vi "P2_Contador99.vi"() -> ()   [LabVIEW 2020]
panel:
  out "a 2":bool
  out "f":bool
  out "e":bool
  out "b":bool
  out "a":bool
  out "b 2":bool
  out "c 2":bool
  out "d 2":bool
  out "g 2":bool
  out "f 2":bool
  out "e 2":bool
  out "c":bool
  out "d":bool
  out "g":bool
  in  "?":bool
  in  "?":bool
  # "Ascendente"
  # "Descendente"
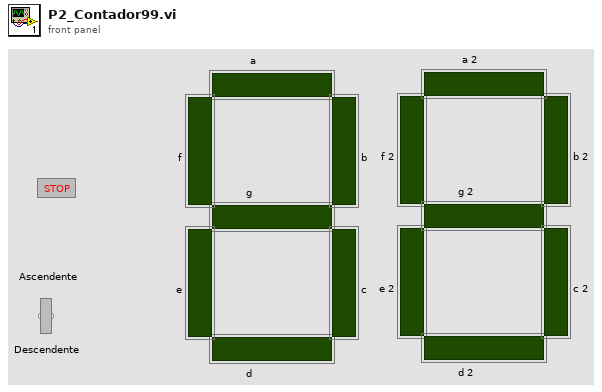
[diagram p1: front panel]
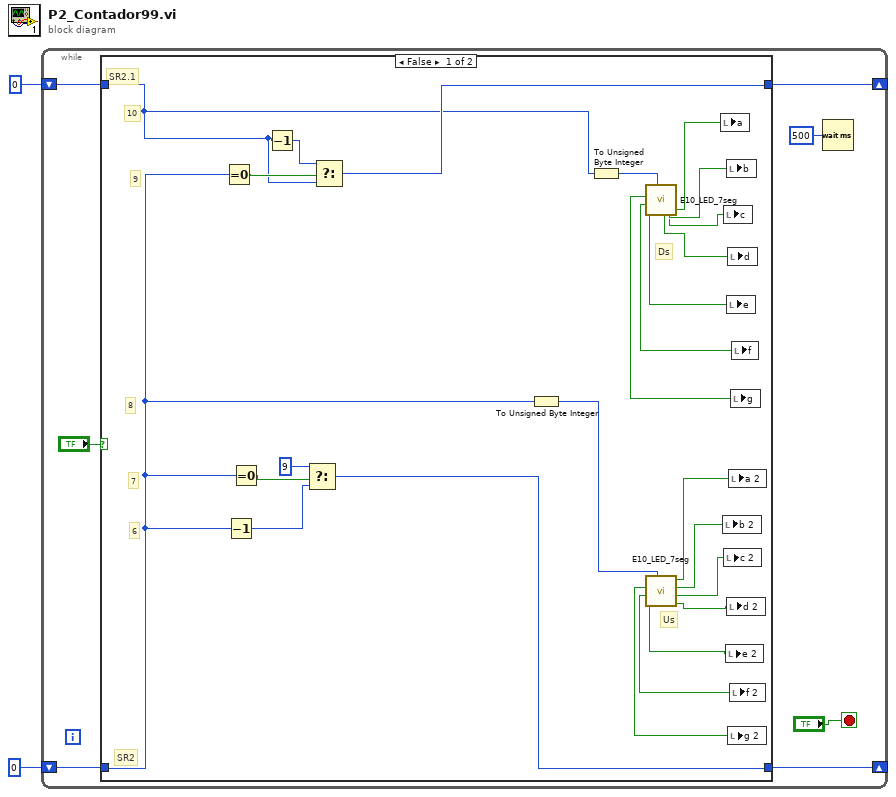
[diagram p0: block diagram]
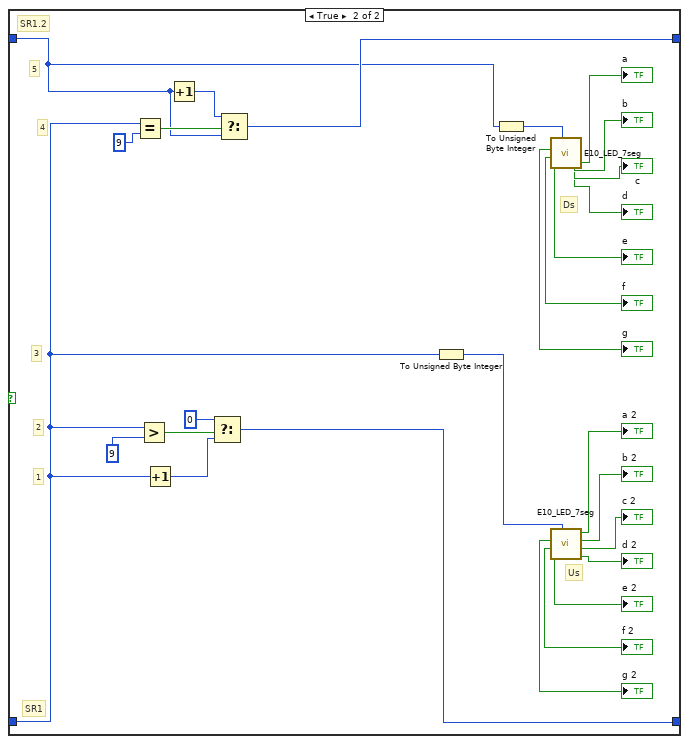
[diagram p2: hidden frame]
diagram:
  n1 = while {
    shift-right: [w8] -> _
    shift-left: 0 -> [w7]
    shift-right: [w5] -> _
    shift-left: 0 -> [w6]
    stop <- "?" stop-if-true
    n2 = case shown="False" "?" {
      tunnel: [w31 w44] -> w8
      tunnel: w7 -> [w11 w37]
      tunnel: w6 -> [w10 w35]
      tunnel: [w13 w36] -> w5
      frame False {
        # "SR2.1"
        # "SR2"
        # "10"
        # "9"
        # "8"
        # "7"
        # "6"
        # "Ds"
        # "Us"
        n3 = Equal To 0?(x=w11) -> (x = 0?=w29:bool)
        n4 = Decrement(x=w11) -> (x-1=w28:i32)
        n5 = Equal To 0?(x=w11) -> (x = 0?=w30:bool)
        n6 = Decrement(x=w10) -> (x-1=w12:i32)
        n7 = Select(t=9, s=w30, f=w28) -> (s? t:f=w31:i32)
        n8 = Select(t=w12, s=w29, f=w10) -> (s? t:f=w13:i32)
        n9 = To Unsigned Byte Integer(number=w11) -> (unsigned 8bit integer=w33:u8)
        n10 = To Unsigned Byte Integer(number=w10) -> (unsigned 8bit integer=w34:u8)
        n11 = call "E10_LED_7seg.vi"("Numeric"=w34) -> ("d"=w24:bool, "c"=w25:bool, "b"=w26:bool, "a"=w27:bool, "e"=w23:bool, "f"=w22:bool, "g"=w21:bool)  [unwired: 1 in]
        n12 = call "E10_LED_7seg.vi"("Numeric"=w33) -> ("d"=w17:bool, "c"=w18:bool, "b"=w19:bool, "a"=w20:bool, "e"=w16:bool, "f"=w15:bool, "g"=w14:bool)  [unwired: 1 in]
        n13 = local write "a"(w27) -> ()
        n14 = local write "b 2"(w19) -> ()
        n15 = local write "c"(w25) -> ()
        n16 = local write "c 2"(w18) -> ()
        n17 = local write "e 2"(w16) -> ()
        n18 = local write "b"(w26) -> ()
        n19 = local write "e"(w23) -> ()
        n20 = local write "d 2"(w17) -> ()
        n21 = local write "d"(w24) -> ()
        n22 = local write "g 2"(w14) -> ()
        n23 = local write "a 2"(w20) -> ()
        n24 = local write "f 2"(w15) -> ()
        n25 = local write "g"(w21) -> ()
        n26 = local write "f"(w22) -> ()
      }
      frame True {
        # "SR1.2"
        # "SR1"
        # "5"
        # "4"
        # "3"
        # "2"
        # "1"
        # "Ds"
        # "Us"
        n27 = Equal?(x=w37, y=9) -> (x = y?=w40:bool)
        n28 = Greater?(x=w37, y=9) -> (0:w45:bool)
        n29 = Increment(x=w37) -> (x+1=w47:i32)
        n30 = Increment(x=w35) -> (x+1=w39:i32)
        n31 = Select(t=0, s=w45, f=w47) -> (s? t:f=w44:i32)
        n32 = Select(t=w39, s=w40, f=w35) -> (s? t:f=w36:i32)
        n33 = To Unsigned Byte Integer(number=w37) -> (unsigned 8bit integer=w42:u8)
        n34 = To Unsigned Byte Integer(number=w35) -> (unsigned 8bit integer=w43:u8)
        n35 = call "E10_LED_7seg.vi"("Numeric"=w43) -> ("d"=→"d":bool, "c"=→"c":bool, "b"=→"b":bool, "a"=→"a":bool, "e"=→"e":bool, "f"=→"f":bool, "g"=→"g":bool)  [unwired: 1 in]
        n36 = call "E10_LED_7seg.vi"("Numeric"=w42) -> ("d"=→"d 2":bool, "c"=→"c 2":bool, "b"=→"b 2":bool, "a"=→"a 2":bool, "e"=→"e 2":bool, "f"=→"f 2":bool, "g"=→"g 2":bool)  [unwired: 1 in]
      }
    }
    n37 = Wait (ms)(milliseconds to wait=u32 500) -> ()  [unwired: 1 out]
  }
